vi "Add Description Values.vi"(8 "error in (no error)":errorcluster, 9 "Release Notes":string, 10 "Description":string, 11 "Map in":map{string, string}(c390)) -> (0 "error out":errorcluster, 3 "Map out":map{string, string}(c390))   [LabVIEW 2019, in "NIPKG Packager.lvclass"]
uses:
  NIPKG Packager.lvclass
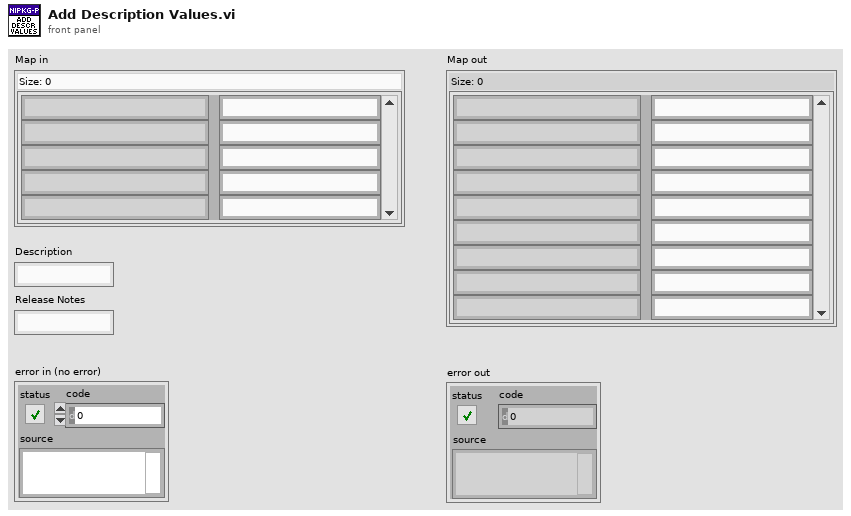
[diagram p1: front panel]
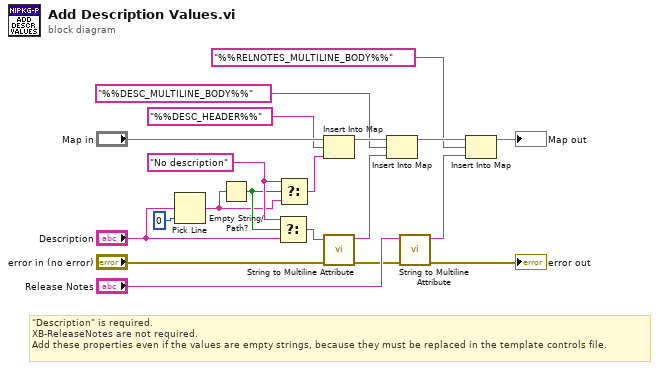
[diagram p0: block diagram]
diagram:
  w20 = "No description" ("t")
  # "\"Description\" is required.\nXB-ReleaseNotes are not required.\nAdd these properties even if the values are empty strings, because they must be replaced in the template controls file."
  n1 = Pick Line(multi-line string="Description", line index=0) -> (output string=w3:string)  [unwired: 1 in]
  n2 = Empty String/Path?(string/path=w3) -> (empty?=w4:bool)
  n3 = Select(t=w20, s=w4, f="Description") -> (s? t:f=w1:string)
  n4 = Select(t=w20, s=w4, f=w3) -> (s? t:f=w5:string)
  n5 = Insert Into Map(map in="Map in", key="%%DESC_HEADER%%", value=w5) -> (map out=w18:map{string, string})  [unwired: 2 out]
  n6 = call "String to Multiline Attribute.vi"("error in (no error)"="error in (no error)", "Multiline String"=w1) -> ("error out"=w7:errorcluster, "Multiline Attribute"=w9:string)  [unwired: 8 in]
  n7 = Insert Into Map(map in=w18, key="%%DESC_MULTILINE_BODY%%", value=w9) -> (map out=w17:map{string, string})  [unwired: 2 out]
  n8 = call "String to Multiline Attribute.vi"("error in (no error)"=w7, "Multiline String"="Release Notes") -> ("error out"=→"error out":errorcluster, "Multiline Attribute"=w10:string)  [unwired: 8 in]
  n9 = Insert Into Map(map in=w17, key="%%RELNOTES_MULTILINE_BODY%%", value=w10) -> (map out=→"Map out":map{string, string})  [unwired: 2 out]
